vi "Create image instace for IP.vi"() -> (1 "bin":T1, 2 "Zoom":T1, 3 "algo2":T1)   [LabVIEW 2015]
uses:
  <vilib>/vision/Image Controls.llb/IMAQ Image.ctl
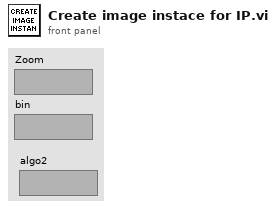
[diagram p1: front panel]
types:
  T1 = typedef "IMAQ Image.ctl" = refnum<image>
  T2 = typedef "Image Type" = u32
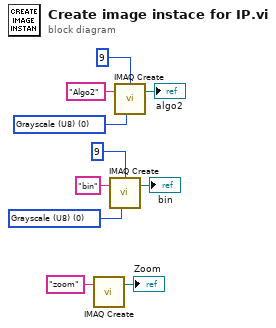
[diagram p0: block diagram]
diagram:
  w7 = T2 0 items=["Grayscale (U8)", "Grayscale (I16)", "Grayscale (SGL)", "Complex (CSG)", "RGB (U32)", "HSL (U32)", "RGB (U64)", "Grayscale (U16)"] ("Image Type")
  w10 = T2 0 items=["Grayscale (U8)", "Grayscale (I16)", "Grayscale (SGL)", "Complex (CSG)", "RGB (U32)", "HSL (U32)", "RGB (U64)", "Grayscale (U16)"] ("Image Type")
  n1 = call "IMAQ Create"("Image Name"="zoom") -> ("New Image"=→"Zoom":T1)  [unwired: 3 in, 2 out]
  n2 = call "IMAQ Create"("Border Size"=9, "Image Name"="bin", "Image Type"=w7) -> ("New Image"=→"bin":T1)  [unwired: 2 in, 1 out]
  n3 = call "IMAQ Create"("Border Size"=9, "Image Name"="Algo2", "Image Type"=w10) -> ("New Image"=→"algo2":T1)  [unwired: 2 in, 1 out]
